vi "Laborator3 (String).vi"() -> ()   [LabVIEW 2023]
panel:
  out "Nr. caractere":i32
  out "Prenume si Nume":string
  in  "Prenume":string
  in  "Nume":string
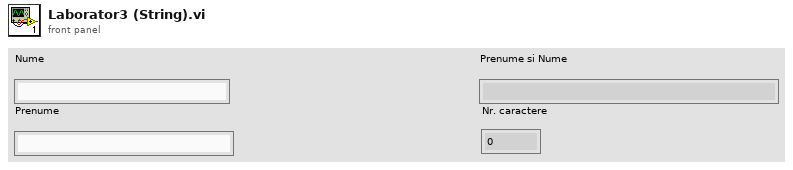
[diagram p1: front panel]
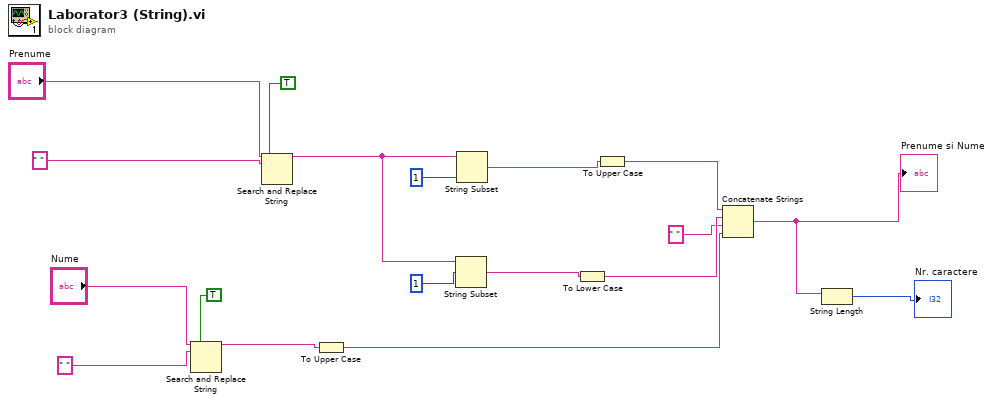
[diagram p0: block diagram]
diagram:
  n1 = Search and Replace String(replace all?=TRUE, input string="Nume", search string=" ") -> (result string=w7:string)  [unwired: 5 in, 3 out]
  n2 = Search and Replace String(replace all?=TRUE, input string="Prenume", search string=" ") -> (result string=w15:string)  [unwired: 5 in, 3 out]
  n3 = To Upper Case(1:w7) -> (0:w4:string)
  n4 = String Subset(string=w15, offset (0)=1) -> (substring=w11:string)  [unwired: 1 in]
  n5 = String Subset(string=w15, length (rest)=1) -> (substring=w12:string)  [unwired: 1 in]
  n6 = To Lower Case(string=w11) -> (all lower case string=w5:string)
  n7 = To Upper Case(1:w12) -> (0:w6:string)
  n8 = Concatenate Strings(w6, w5, " ", w4) -> (w3:string)
  "Prenume si Nume" <- w3
  n9 = String Length(string=w3) -> (length=→"Nr. caractere":i32)
